vi "Get Object.vi"(8 "error in":errorcluster, 9 "Sub-Index":i16=-1, 10 "Index":u16 format="%04x", 11 "EDS in":refnum<class "EDS.lvclass">) -> (0 "error out":errorcluster, 1 "OD Entry":refnum<class "OD Entry.lvclass">, 2 "Found?":bool, 3 "EDS out":refnum<class "EDS.lvclass">)   [LabVIEW 2024, in "EDS.lvlib" / "EDS.lvclass"]
uses:
  EDS.lvclass
  OD Entry/OD Entry.lvclass
  EDS.lvclass/EDS.ctl
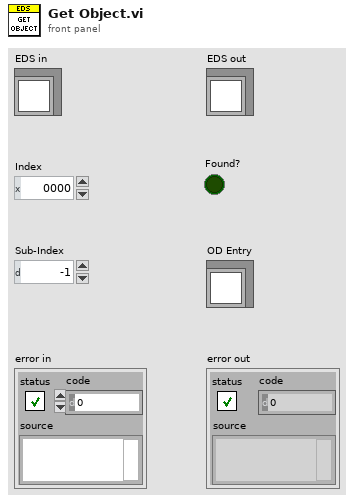
[diagram p1: front panel]
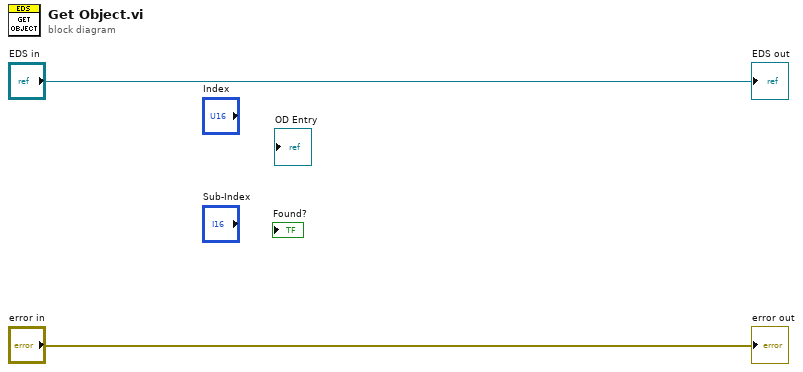
[diagram p0: block diagram]
diagram:
  "error out" <- "error in"
  "EDS out" <- "EDS in"
